vi "empty tube.vi"() -> ()   [LabVIEW 2013]
uses:
  <vilib>/DAQmx/read.llb/DAQmx Read (Digital 1D U8 1Chan NSamp).vi
  <vilib>/DAQmx/write.llb/DAQmx Write (Digital Bool 1Line 1Point).vi
  <vilib>/DAQmx/create/channels.llb/DAQmx Create Channel (DO-Digital Output).vi
  <vilib>/DAQmx/create/channels.llb/DAQmx Create Channel (DI-Digital Input).vi
  <vilib>/DAQmx/configure/timing.llb/DAQmx Timing (Sample Clock).vi
  <vilib>/DAQmx/miscellaneous.llb/DAQmx Fill In Error Info.vi
  <vilib>/Analysis/NI_AALBase.lvlib
panel:
  out "Green Light":bool
  out "click time":u32
  in  "lick sample rate":dbl=500.0 format="%#_13g"
  out "Lick Detection":dbl[](graph)
  in  "milliseconds to wait":u32=200
  in  "Click":bool
  in  "stop":bool
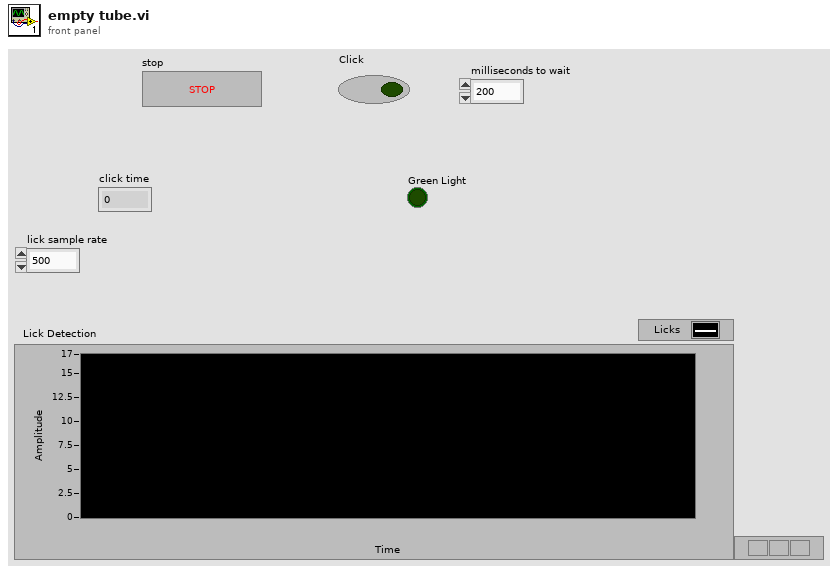
[diagram p1: front panel]
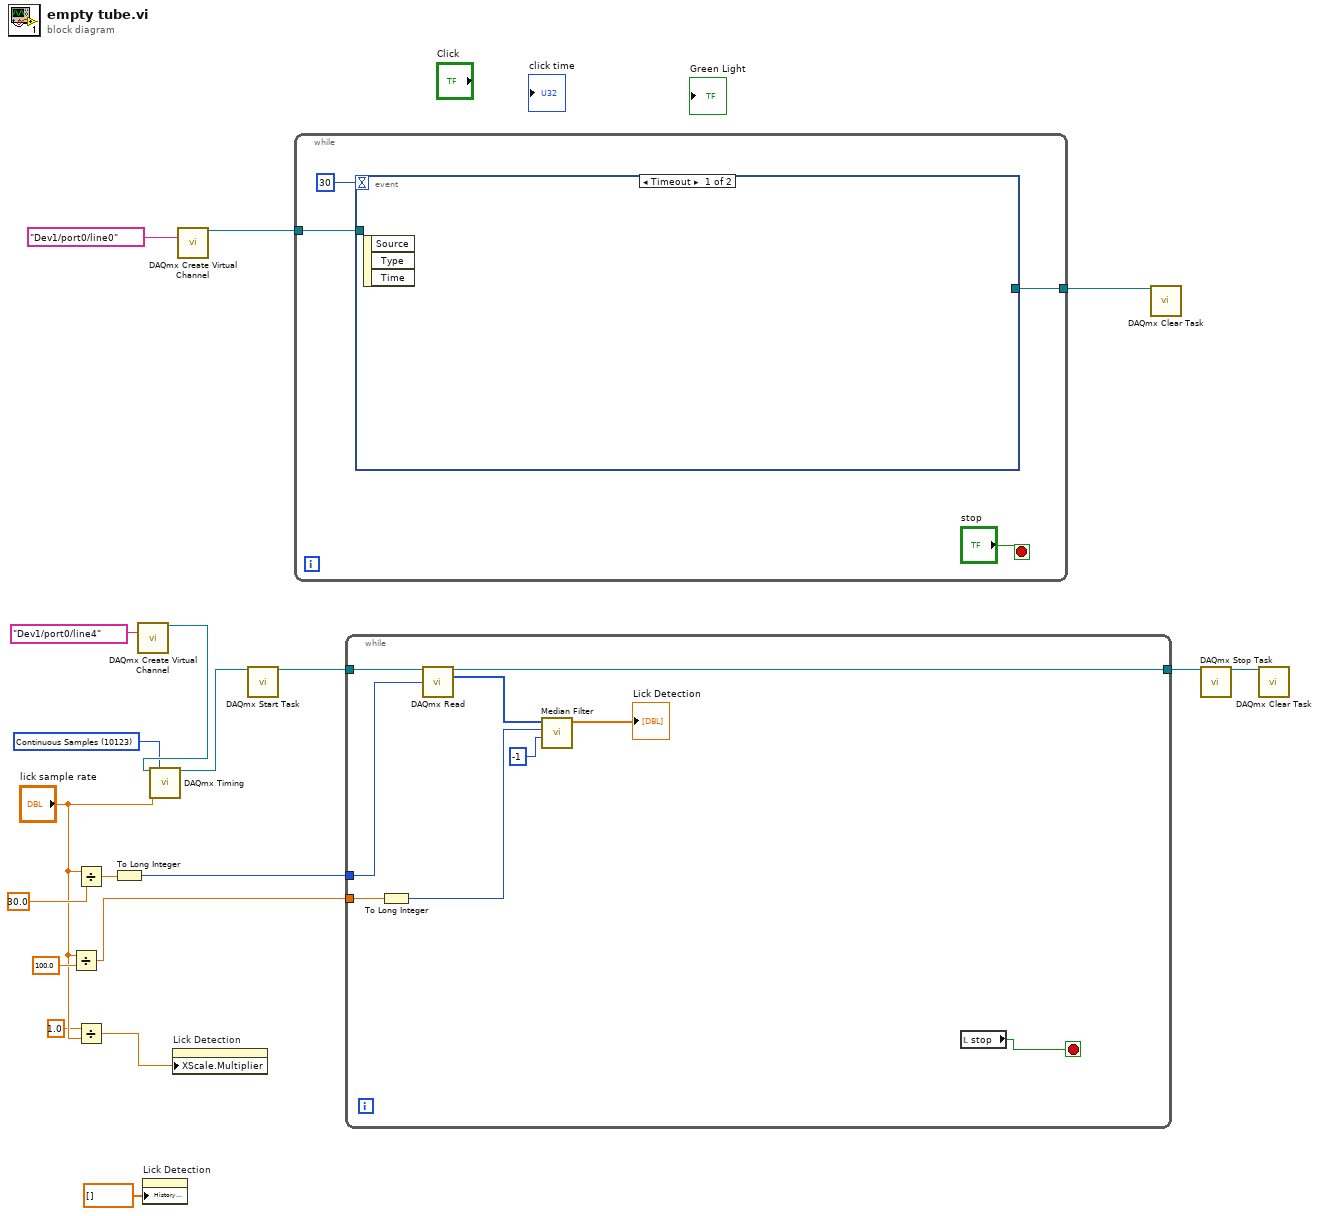
[diagram p0: block diagram]
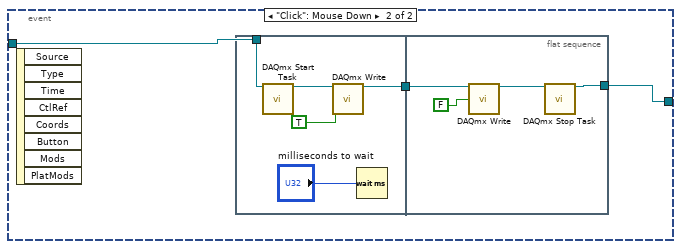
[diagram p2: hidden frame]
diagram:
  w10 = 10123 items=["Finite Samples"=10178, "Continuous Samples"=10123, "Hardware Timed Single Point"=12522] ("sample mode")
  n1 = Divide(x="lick sample rate", y=100.0) -> (x/y=w5:dbl)
  n2 = Divide(x="lick sample rate", y=30.0) -> (x/y=w9:dbl)
  n3 = Divide(x=1.0, y="lick sample rate") -> (x/y=w2:dbl)
  n4 = To Long Integer(number=w9) -> (32bit integer=w7:i32)
  n5 = call-poly <vilib>:"DAQmx Create Virtual Channel.vi"("lines"=tag "Dev1/port0/line4" ("lick detection")) -> ("task out"=w12:refnum<k21>)  [unwired: 13 in, 1 out]
  n6 = property on="Lick Detection" class="WFChart (strict)"("History Data"=dbl[] []) -> ()  [unwired: 2 in, 2 out]
  n7 = call-poly <vilib>:"DAQmx Timing.vi"("task/channels in"=w12, "sample mode"=w10, "rate"="lick sample rate") -> ("task out"=w11:refnum<k21>)  [unwired: 11 in, 1 out]
  n8 = property on="Lick Detection" class="WFChart (strict)"("XScale.Multiplier"=w2) -> ()  [unwired: 2 in, 2 out]
  n9 = call-poly <vilib>:"DAQmx Create Virtual Channel.vi"("lines"=tag "Dev1/port0/line0") -> ("task out"=w18:refnum<k21>)  [unwired: 13 in, 1 out]
  n10 = call <vilib>:"DAQmx Start Task.vi"("task/channels in"=w11) -> ("task out"=w15:refnum<k21>)  [unwired: 13 in, 1 out]
  n11 = while {
    tunnel: w18 -> [w23]
    tunnel: [w22] -> w17
    stop <- "stop" stop-if-true
    n12 = event shown="[0] Timeout" {
      selector: _ -> [_ _]
      dyn-events: _ -> [_ _]
      timeout: 30 -> [_ _]
      tunnel: w23 -> [_ w26]
      tunnel: [_ w25] -> w22
      event Timeout {
        n13 = event-data() -> ()  [unwired: 1 in, 3 out]
      }
      event "Click": Mouse Down {
        n14 = event-data() -> ()  [unwired: 1 in, 8 out]
        n15 = flat-sequence {
          tunnel: w26 -> [w31]
          tunnel: [w28] -> w24
          tunnel: w24 -> [w35]
          tunnel: [w32] -> w25
          frame #0 {
            n16 = call <vilib>:"DAQmx Start Task.vi"("task/channels in"=w31) -> ("task out"=w29:refnum<k21>)  [unwired: 13 in, 1 out]
            n17 = call-poly <vilib>:"DAQmx Write.vi"("task/channels in"=w29, "data"=TRUE) -> ("task out"=w28:refnum<k21>)  [unwired: 11 in, 2 out]
            n18 = Wait (ms)(milliseconds to wait="milliseconds to wait") -> ()  [unwired: 1 out]
          }
          frame #1 {
            n19 = call-poly <vilib>:"DAQmx Write.vi"("task/channels in"=w35, "data"=FALSE) -> ("task out"=w34:refnum<k21>)  [unwired: 11 in, 2 out]
            n20 = call <vilib>:"DAQmx Stop Task.vi"("task/channels in"=w34) -> ("task out"=w32:refnum<k21>)  [unwired: 13 in, 1 out]
          }
        }
      }
    }
  }
  n21 = while {
    tunnel: w15 -> [w44]
    tunnel: [w43] -> w14
    tunnel: w7 -> [w40]
    tunnel: w5 -> [w39]
    stop <- w36 stop-if-true
    n22 = To Long Integer(number=w39) -> (32bit integer=w38:i32)
    n23 = call-poly <vilib>:"DAQmx Read.vi"("task/channels in"=w44, "number of samples per channel"=w40) -> ("task out"=w43:refnum<k21>, "data"=w42:u8[])  [unwired: 11 in, 1 out]
    n24 = call <vilib>:"Median Filter.vi"("right rank"=-1, "left rank"=w38, "X"=w42) -> ("Filtered X"=→"Lick Detection":dbl[])  [unwired: 7 in, 1 out]
    n25 = local read "stop"() -> (w36:bool)
  }
  n26 = call <vilib>:"DAQmx Clear Task.vi"("task in"=w17) -> ()  [unwired: 14 in, 1 out]
  n27 = call <vilib>:"DAQmx Stop Task.vi"("task/channels in"=w14) -> ("task out"=w13:refnum<k21>)  [unwired: 13 in, 1 out]
  n28 = call <vilib>:"DAQmx Clear Task.vi"("task in"=w13) -> ()  [unwired: 14 in, 1 out]
